vi "TSC_Query.vi"(0 "System no.":i32=1 min=1 max=4 step=1, 5 "error in":errorcluster) -> (14 "Number of sensor channels":i32, 19 "error out":errorcluster)   [LabVIEW 2020]
doc: "Returns the number of available sensor channels. \n\nE-517: Using the Sensor Enable parameter, ID 0x02000000, you can change the E-517 configuration in case of hardware changes, e.g. if you install additional sensor and/or amplifier channels in the system. If this parameter is changed, the Number Of Sensor Channels parameter is adapted automatically. E.g. if parameter 0x02000000 is set to \"disabled\" for a sensor channel, this sensor channel is no longer included in the TSC? response. See \"Configure Axes and Channels\" in the E-517 User manual for details.\n\nE-709: The response comprises all ADC channels of the device: the \"genuine\" sensor (sensor integrated in the mechanics) and the \"general purpose\" analog input.\n\nC-413, E-712, E-725, E-727: The response comprises all ADC channels of the device: \"genuine\" sensors (sensors integrated in the mechanics) and \"general purpose\" analog input channels.\n\nE-753: The response comprises all ADC channels of the device: the \"genuine\" sensor (capacitive sensor integrated in the mechanics) and the \"general purpose\" analog input.\nE-754: The response comprises all ADC channels of the device: the \"genuine\" sensor (capacitive or incremental sensors integrated in the mechanics) and the \"general purpose\" analog input."
panel:
  # "Returns the number of available sensor channels."
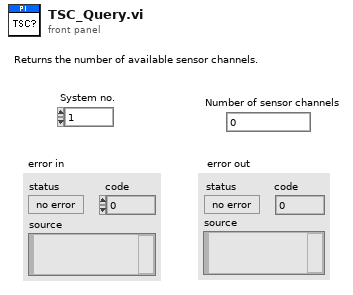
[diagram p1: front panel]
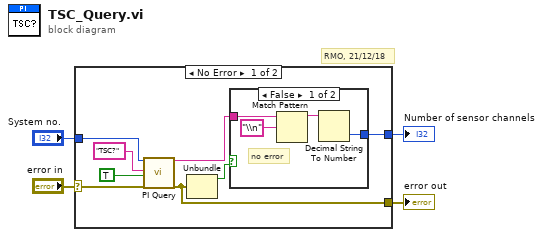
[diagram p0: block diagram]
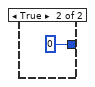
[diagram p2: hidden frame]
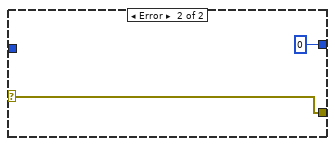
[diagram p3: hidden frame]
diagram:
  # "RMO, 21/12/18"
  n1 = case shown="No Error" "error in" {
    selector: "error in" -> [w7 w19]
    tunnel: [w11 0] -> w4
    tunnel: [w6 w19] -> w3
    tunnel: "System no." -> [w9 _]
    frame No Error {
      n2 = call "PI Query.vi"("System no."=w9, "String to send"="TSC?", "Attach termination char.?"=TRUE ("Attach Linefeed?"), "error in"=w7) -> ("String read"=w5:string, "error out"=w6:errorcluster)  [unwired: 3 in, 11 out]
      n3 = Unbundle(w6) -> ("status"=w12:bool)  [unwired: 2 out]
      n4 = case shown="False" w12 {
        tunnel: w5 -> [w15 _]
        tunnel: [w16 0] -> w11
        frame False {
          # "no error"
          n5 = Match Pattern(string=w15, regular expression="\\n") -> (before substring=w13:string)  [unwired: 4 out]
          n6 = Decimal String To Number(string=w13) -> (number=w16:i32)  [unwired: 3 out]
        }
        frame True {
        }
      }
    }
    frame Error {
    }
  }
  "error out" <- w3
  "Number of sensor channels" <- w4
